vi "set Data Element.vi"(0 "LVx - Template Command in":refnum<class "REx - NART - Report Calibration Point Power.lvclass">, 5 "Power, dB":dbl=62.0, 11 "error in (no error)":errorcluster) -> (4 "LVx - Template Command out":refnum<class "REx - NART - Report Calibration Point Power.lvclass">, 15 "error out":errorcluster)   [LabVIEW 2011, in "ART2 Test Panel.lvlib" / "REx - NART - Report Calibration Point Power.lvclass"]
uses:
  REx - NART - Calibrate/REx - NART - Report Calibration Point Power.lvclass
  REx - NART - Calibrate/REx - NART - Report Calibration Point Power.lvclass/REx - NART - Report Calibration Point Power.ctl
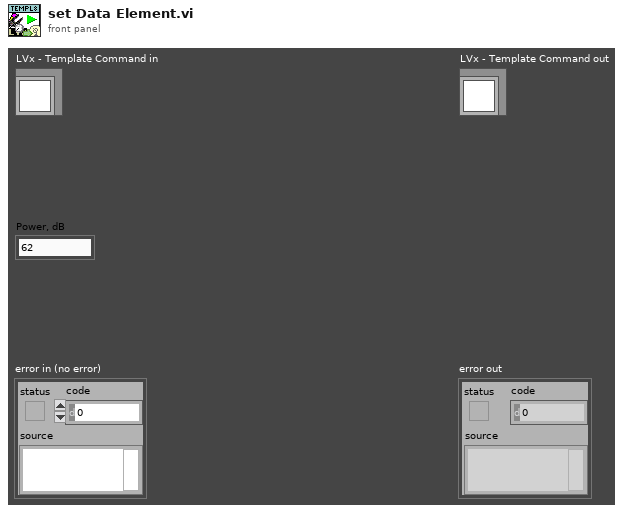
[diagram p1: front panel]
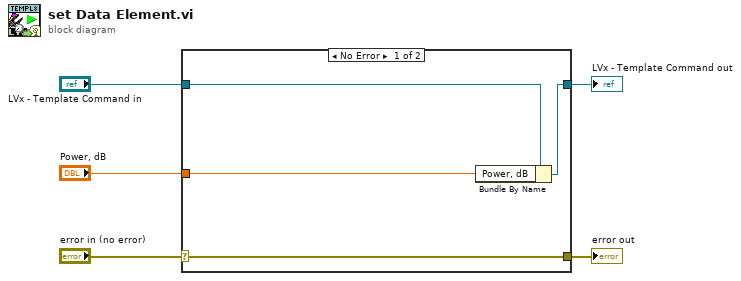
[diagram p0: block diagram]
diagram:
  n1 = case shown="No Error" "error in (no error)" {
    selector: "error in (no error)" -> [w9 w10]
    tunnel: [w9 w10] -> w4
    tunnel: [w7 w11] -> w2
    tunnel: "LVx - Template Command in" -> [w8 w11]
    tunnel: "Power, dB" -> [w6 _]
    frame No Error {
      n2 = Bundle By Name(cluster=w8, "Power, dB"=w6) -> (w7:refnum<class "REx - NART - Report Calibration Point Power.lvclass">)
    }
    frame Error {
    }
  }
  "error out" <- w4
  "LVx - Template Command out" <- w2
